vi "Configure Zeroing.vi"(0 "VISA resource name":refnum<visa-resource-name>, 5 "Autozero (T: Enable)":bool=TRUE, 7 "Enable Zero Correct (F: Disable)":bool, 11 "error in (no error)":errorcluster) -> (4 "VISA resource name out":refnum<visa-resource-name>, 15 "error out":errorcluster)   [LabVIEW 2020, in "Keithley 648X Series.lvlib"]
doc: "Enables or disables the autozero and zero correct functionalities.\n\n<b>Note:</b>\nTo acquire a zero correct value use the <b>Acquire Zero Correct</b> action VI."
uses:
  <instrlib>/Keithley 648X Series/Keithley 648X Series.lvlib
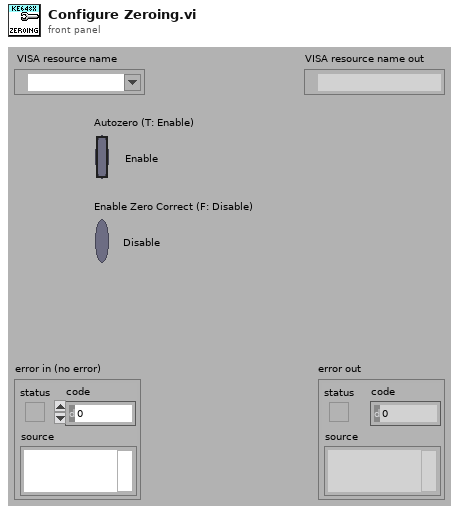
[diagram p1: front panel]
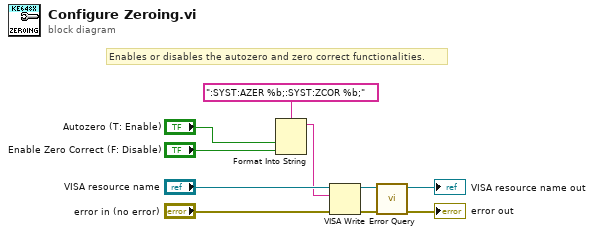
[diagram p0: block diagram]
diagram:
  # "Enables or disables the autozero and zero correct functionalities."
  n1 = Format Into String(format string=":SYST:AZER %b;:SYST:ZCOR %b;", "Autozero (T: Enable)", "Enable Zero Correct (F: Disable)") -> (resulting string=w2:string)  [unwired: 2 in, 1 out]
  n2 = VISA Write(VISA resource name="VISA resource name", write buffer=w2, error in (no error)="error in (no error)") -> (VISA resource name out=w6:refnum<visa-resource-name>, error out=w5:errorcluster)  [unwired: 1 out]
  n3 = call <instrlib>:"Error Query.vi"("error in (no error)"=w5, "VISA resource name"=w6) -> ("error out"=→"error out":errorcluster, "VISA resource name out"=→"VISA resource name out":refnum<visa-resource-name>)  [unwired: 6 in, 2 out]
